vi "EdgeOff.vi"(11 "Input":bool) -> (3 "Edge Off":bool)   [LabVIEW 2020]
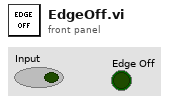
[diagram p1: front panel]
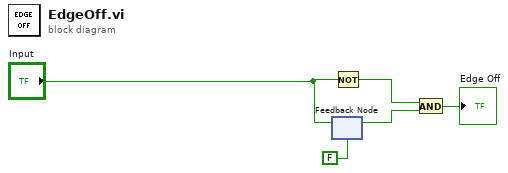
[diagram p0: block diagram]
diagram:
  n1 = feedback #1(FALSE ("Capture Cube")) -> (w1:bool)
  n2 = feedback-in #1("Input") -> ()
  n3 = Not(x="Input") -> (.not. x?=w2:bool)
  n4 = And(x=w2, y=w1) -> (x .and. y?=→"Edge Off":bool)
